vi "Signal Input.vi"(8 "error in (no error)":errorcluster) -> (0 "error out":errorcluster)   [LabVIEW 2019, in "Haptic Prog Interface.lvlib"]
doc: "Returns the forces of the haptic pen in N.\n\n<b>Position:</b> Returns a cluster of the x, y, and z forces on the pen (in units of N)."
uses:
  Haptic Prog Interface.lvlib
  dll_path.vi
panel:
  in  "Gain":dbl=1.0 format="%_2p"
  in  "Signal":dbl format="%_2p"
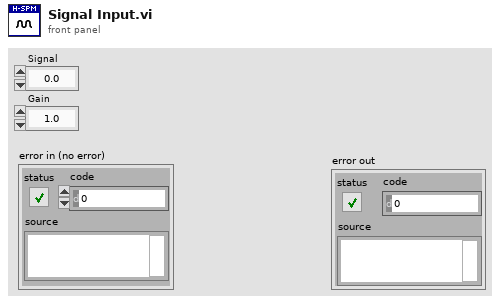
[diagram p1: front panel]
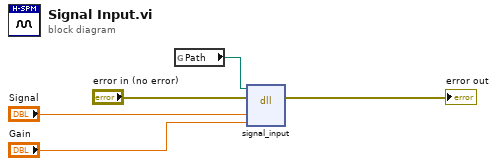
[diagram p0: block diagram]
diagram:
  n1 = global read "dll_path.vi" "Path"() -> (w5:path)
  n2 = dll-call lib="C:/Users/freem/Documents/GitHub/HapticSPM/Haptic-Programming-Interface/x64/Debug/Haptic Programming Interface.dll" fn="signal_input"(path in=w5, error in="error in (no error)", "input_signal"="Signal", "input_gain"="Gain") -> (error out=→"error out":errorcluster)  [unwired: 4 in, 1 out]
